vi "control_lasers_and_SMs_wavelength_5s_alts.vi"() -> ()   [LabVIEW 2021]
uses:
  <vilib>/DAQmx/create/channels.llb/DAQmx Create Channel (AO-Voltage-Basic).vi
  <vilib>/DAQmx/write.llb/DAQmx Write (Analog 1D DBL NChan 1Samp).vi
  <vilib>/DAQmx/write.llb/DAQmx Write (Analog DBL 1Chan 1Samp).vi
panel:
  in  "Y2":dbl
  in  "X2":dbl
  in  "Y1 (-10-10V)":dbl
  in  "X1 (-10-10V)":dbl
  in  "Blanking (0-10v)":dbl=10.0
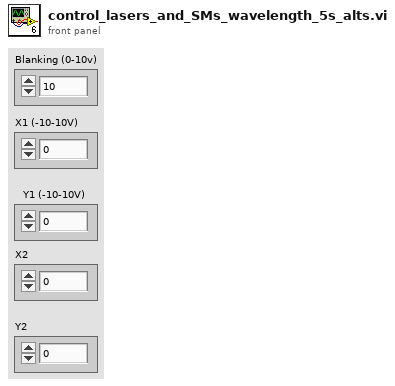
[diagram p1: front panel]
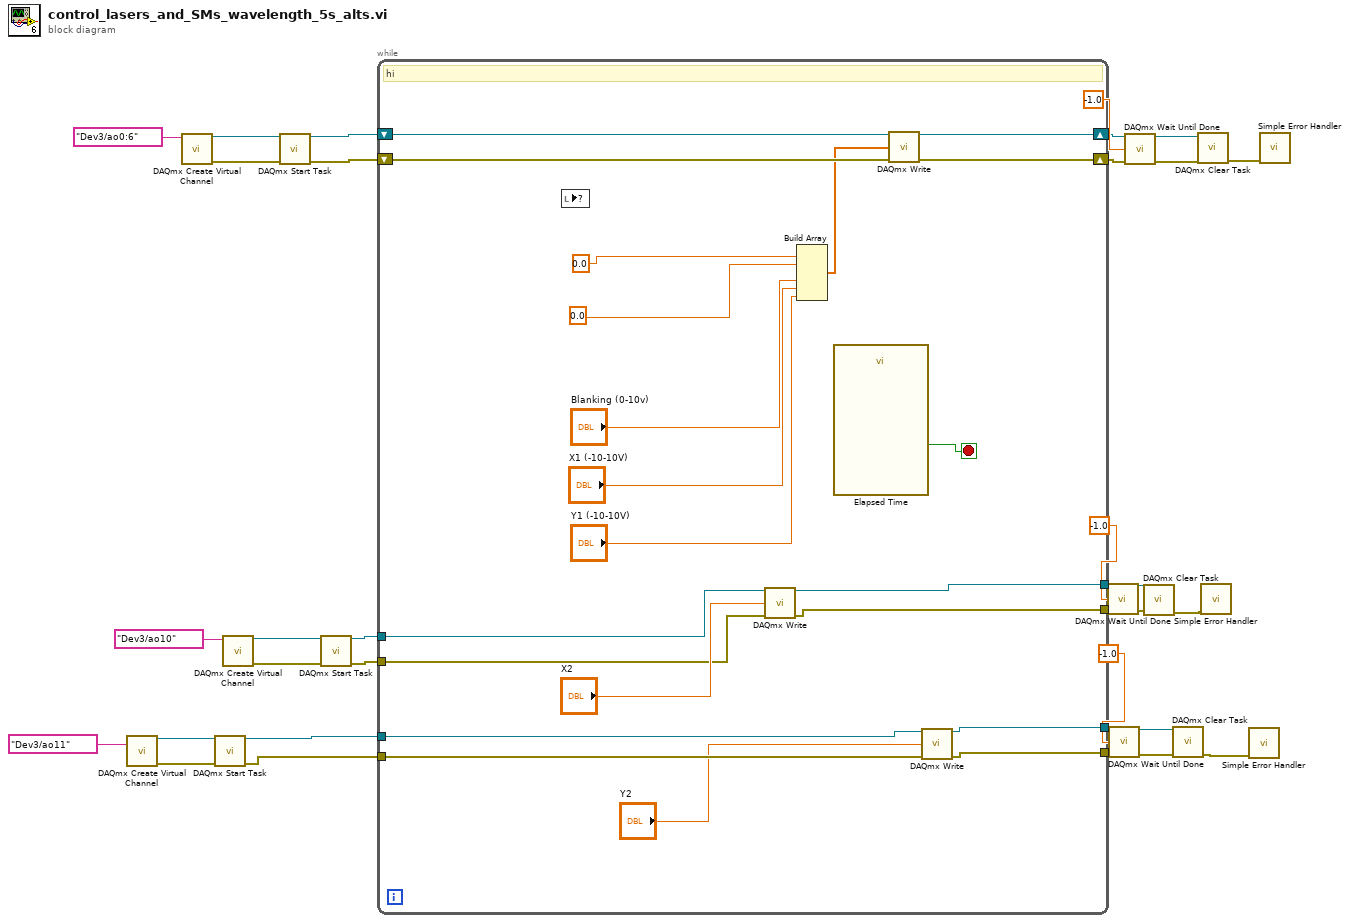
[diagram p0: block diagram]
diagram:
  n1 = call-poly <vilib>:"DAQmx Create Virtual Channel.vi"("physical channels"=tag "Dev3/ao11") -> ("task out"=w10:refnum<k21>, "error out"=w9:errorcluster)  [unwired: 13 in]
  n2 = call-poly <vilib>:"DAQmx Create Virtual Channel.vi"("physical channels"=tag "Dev3/ao0:6") -> ("task out"=w26:refnum<k21>, "error out"=w25:errorcluster)  [unwired: 13 in]
  n3 = call <vilib>:"DAQmx Start Task.vi"("task/channels in"=w10, "error in"=w9) -> ("task out"=w7:refnum<k21>, "error out"=w8:errorcluster)  [unwired: 12 in]
  n4 = call-poly <vilib>:"DAQmx Create Virtual Channel.vi"("physical channels"=tag "Dev3/ao10") -> ("task out"=w21:refnum<k21>, "error out"=w20:errorcluster)  [unwired: 13 in]
  n5 = call <vilib>:"DAQmx Start Task.vi"("task/channels in"=w26, "error in"=w25) -> ("task out"=w28:refnum<k21>, "error out"=w27:errorcluster)  [unwired: 12 in]
  n6 = call <vilib>:"DAQmx Start Task.vi"("task/channels in"=w21, "error in"=w20) -> ("task out"=w16:refnum<k21>, "error out"=w15:errorcluster)  [unwired: 12 in]
  n7 = while {
    shift-right: [w53] -> w23
    shift-left: w28 -> [w55]
    shift-right: [w52] -> w24
    shift-left: w27 -> [w54]
    tunnel: w16 -> [w47]
    tunnel: w15 -> [w45]
    tunnel: [w44] -> w14
    tunnel: [w43] -> w13
    tunnel: w8 -> [w42]
    tunnel: w7 -> [w40]
    tunnel: [w39] -> w4
    tunnel: [w38] -> w3
    stop <- w34 stop-if-true
    # "hi"
    n8 = local read item#-1() -> ()  [unwired: 1 in]
    n9 = call-poly <vilib>:"DAQmx Write.vi"("task/channels in"=w47, "data"="X2", "error in"=w45) -> ("task out"=w44:refnum<k21>, "error out"=w43:errorcluster)  [unwired: 10 in, 1 out]
    n10 = Build Array(0.0, 0.0 ("element"), "Blanking (0-10v)", "X1 (-10-10V)", "Y1 (-10-10V)") -> (w51:dbl[], w36:dbl)  [unwired: 1 in]
    n11 = call "Elapsed Time"() -> ("Time has Elapsed"=w34:bool)  [unwired: 12 in, 7 out]
    n12 = call-poly <vilib>:"DAQmx Write.vi"("task/channels in"=w55, "data"=w51, "error in"=w54) -> ("task out"=w53:refnum<k21>, "error out"=w52:errorcluster)  [unwired: 10 in, 1 out]
    n13 = call-poly <vilib>:"DAQmx Write.vi"("task/channels in"=w40, "data"="Y2", "error in"=w42) -> ("task out"=w39:refnum<k21>, "error out"=w38:errorcluster)  [unwired: 10 in, 1 out]
  }
  n14 = call <vilib>:"DAQmx Wait Until Done.vi"("task/channels in"=w14, "timeout (sec)"=-1.0, "error in"=w13) -> ("task out"=w18:refnum<k21>, "error out"=w17:errorcluster)  [unwired: 11 in]
  n15 = call <vilib>:"DAQmx Wait Until Done.vi"("task/channels in"=w4, "timeout (sec)"=-1.0, "error in"=w3) -> ("task out"=w1:refnum<k21>, "error out"=w2:errorcluster)  [unwired: 11 in]
  n16 = call <vilib>:"DAQmx Wait Until Done.vi"("task/channels in"=w23, "timeout (sec)"=-1.0, "error in"=w24) -> ("task out"=w32:refnum<k21>, "error out"=w31:errorcluster)  [unwired: 11 in]
  n17 = call <vilib>:"DAQmx Clear Task.vi"("task in"=w18, "error in"=w17) -> ("error out"=w19:errorcluster)  [unwired: 13 in]
  n18 = call <vilib>:"DAQmx Clear Task.vi"("task in"=w1, "error in"=w2) -> ("error out"=w12:errorcluster)  [unwired: 13 in]
  n19 = call <vilib>:"DAQmx Clear Task.vi"("task in"=w32, "error in"=w31) -> ("error out"=w33:errorcluster)  [unwired: 13 in]
  n20 = call <vilib>:"Simple Error Handler.vi"("error in (no error)"=w19) -> ()  [unwired: 4 in, 5 out]
  n21 = call <vilib>:"Simple Error Handler.vi"("error in (no error)"=w12) -> ()  [unwired: 4 in, 5 out]
  n22 = call <vilib>:"Simple Error Handler.vi"("error in (no error)"=w33) -> ()  [unwired: 4 in, 5 out]
